vi "Draw_Face.vi"(6 "fill?(F)":bool, 9 "color":u32, 10 "Array":cluster{"x":dbl, "y":dbl}[](array[cluster]), 11 "picture in":picture) -> (3 "new picture":picture)   [LabVIEW 2022 SP3]
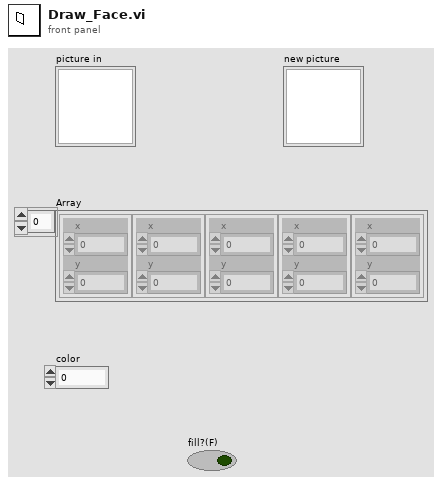
[diagram p1: front panel]
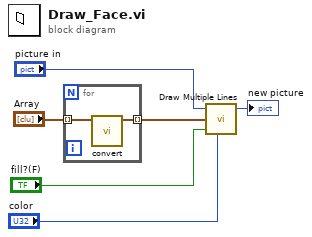
[diagram p0: block diagram]
diagram:
  n1 = for {
    tunnel: "Array" -> [w8] mode=indexing
    tunnel: [w7] -> w1 mode=indexing
    n2 = call "convert.vi"("point"=w8) -> ("scaled"=w7:cluster{"x":dbl, "y":dbl})  [unwired: 10 in]
  }
  n3 = call <vilib>:"Draw Multiple Lines.vi"("picture"="picture in", "line endpoints"=w1, "fill?(F)"="fill?(F)", "color(black)"="color") -> ("new picture"=→"new picture":picture)  [unwired: 5 in]
